vi "getStatus.vi"(0 "reference (in)":refnum<class "_MultiAxisController.lvclass">, 2 "axis":T5, 5 "error in (no error)":errorcluster) -> (14 "reference (out)":refnum<class "_MultiAxisController.lvclass">, 16 "status (raw result)":string, 17 "full_state":T1={"X"={"motion_state"=enum."CONST", "other_states"=[]}, "Y"={"motion_state"=enum."CONST", "other_states"=[]}, "Z"={"motion_state"=enum."CONST", "other_states"=[]}, "U"={"motion_state"=enum."CONST", "other_states"=[]}, "buffer_enabled?"=FALSE, "buffer_start"=0, "buffer_end"=0, "avail_buffer"=0, "move_mode"=enum."ABSOLUTE"}, 19 "error out":errorcluster)   [LabVIEW 2013, in "classes.lvlib" / "_MultiAxisController.lvclass"]
doc: "Produced By:\n\n<B>Kod Integrations, LLC</B>\n4835 Marianne Drive\nMount Airy, MD 21771\nhttp://www.kodintegrations.com\nemail: info@kodintegrations.com\nphone: (240) 687-1288"
uses:
  _MultiAxisController.lvclass
  common/controls/axis.ctl
  common/controls/complete_motor_state.ctl
  common/controls/single_axis_state.ctl
  common/controls/motor_status.ctl
  common/controls/move_mode.ctl
  Controller/_Controller.lvclass
  libraries/common.lvlib
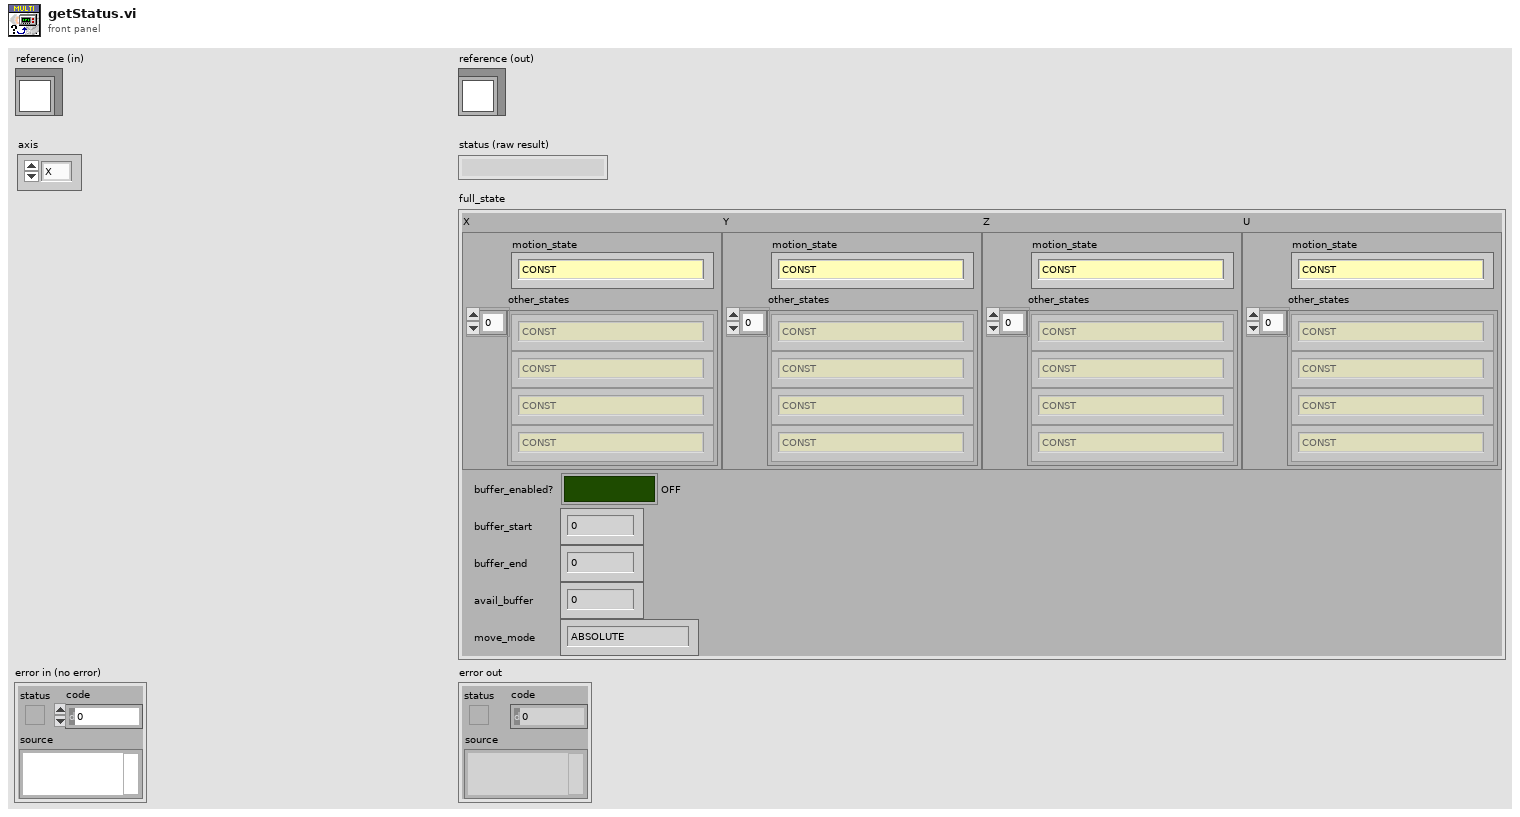
[diagram p1: front panel]
types:
  T1 = typedef "common.lvlib/complete_motor_state.ctl" = cluster{"X":T2, "Y":T2, "Z":T2, "U":T2, "buffer_enabled?":bool, "buffer_start":i32, "buffer_end":i32, "avail_buffer":i32, "move_mode":T4}
  T2 = typedef "common.lvlib/single_axis_state.ctl" = cluster{"motion_state":T3, "other_states":T3[]}
  T3 = typedef "common.lvlib/motor_status.ctl" = enum16{"IDLE", "CONST", "ACCEL", "DECEL", "HOME_SWITCH", "-LIMIT_SWITCH", "+LIMIT_SWITCH", "-LIMIT_ERR", "+LIMIT_ERR", "COMM_TIMEOUT", "ALARM_INPUT", "ALARM_ERROR", "TOC_TIMEOUT_STATUS", "LATCH_INPUT_STATUS", "Z_INDEX_STATUS"}
  T4 = typedef "common.lvlib/move_mode.ctl" = enum16{"ABSOLUTE", "INCREMENTAL"}
  T5 = typedef "common.lvlib/axis.ctl" = enum16{"X", "Y", "Z", "U"}
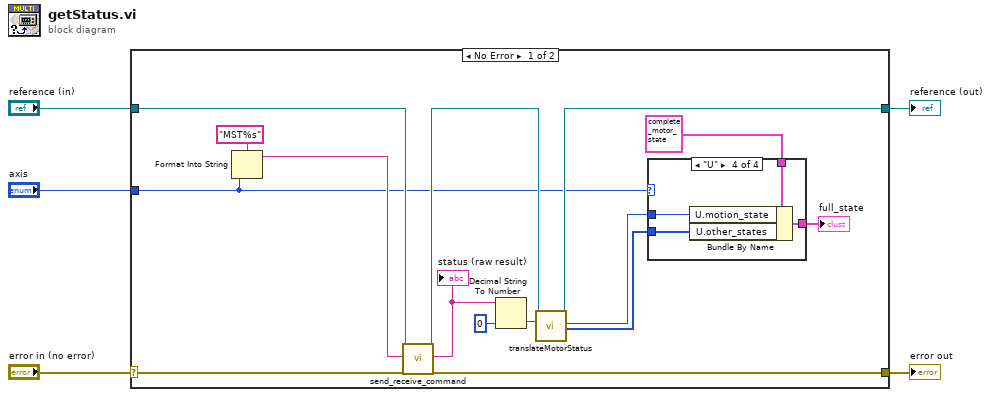
[diagram p0: block diagram]
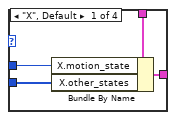
[diagram p2: hidden frame]
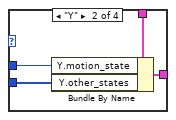
[diagram p3: hidden frame]
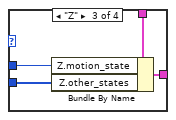
[diagram p4: hidden frame]
diagram:
  n1 = case shown="No Error" "error in (no error)" {
    selector: "error in (no error)" -> [w17 w38]
    tunnel: [w16 w38] -> w4
    tunnel: [w11 w37] -> w2
    tunnel: "reference (in)" -> [w18 w37]
    tunnel: "axis" -> [w9 _]
    frame No Error {
      n2 = Format Into String(format string="MST%s" ("ASCII Command (in)"), w9) -> (resulting string=w14:string)  [unwired: 2 in, 1 out]
      n3 = call "send_receive_command.vi"("reference (in)"=w18, "ASCII Command (in)"=w14, "error in (no error)"=w17) -> ("reference (out)"=w12:refnum<class "_MultiAxisController.lvclass">, "response (out)"=w13:string, "error out"=w16:errorcluster)  [unwired: 12 in, 2 out]
      "status (raw result)" <- w13
      n4 = Decimal String To Number(string=w13, default (0L)=u32 0 ("default (0 I32)")) -> (number=w19:u32)  [unwired: 1 in, 1 out]
      n5 = call-dynamic "translateMotorStatus.vi"("Controller in"=w12, "actual value"=w19) -> ("Controller out"=w11:refnum<class "_MultiAxisController.lvclass">, "motion_state"=w8:T3, "other_states (for use in overiding classes)"=w7:T3[])  [unwired: 14 in, 1 out]
      n6 = case shown="\"U\"" w9 {
        tunnel: T1 {"X"={"motion_state"=enum."IDLE", "other_states"=[]}, "Y"={"motion_state"=enum."IDLE", "other_states"=[]}, "Z"={"motion_state"=enum."IDLE", "other_states"=[]}, "U"={"motion_state"=enum."IDLE", "other_states"=[]}, "buffer_enabled?"=FALSE, "buffer_start"=0, "buffer_end"=0, "avail_buffer"=0, "move_mode"=enum."INCREMENTAL"} ("full_state") -> [w24 w28 w32 w36]
        tunnel: w8 -> [w22 w26 w31 w34]
        tunnel: w7 -> [w21 w25 w30 w33]
        tunnel: [w23 w27 w29 w35] -> w6
        frame "X", Default {
          n7 = Bundle By Name(cluster=w24, "X.motion_state"=w22, "X.other_states"=w21) -> (w23:T1)
        }
        frame "Y" {
          n8 = Bundle By Name(cluster=w28, "Y.motion_state"=w26, "Y.other_states"=w25) -> (w27:T1)
        }
        frame "Z" {
          n9 = Bundle By Name(cluster=w32, "Z.motion_state"=w31, "Z.other_states"=w30) -> (w29:T1)
        }
        frame "U" {
          n10 = Bundle By Name(cluster=w36, "U.motion_state"=w34, "U.other_states"=w33) -> (w35:T1)
        }
      }
      "full_state" <- w6
    }
    frame Error {
    }
  }
  "error out" <- w4
  "reference (out)" <- w2
